vi "ZVisualize.vi"() -> ()   [LabVIEW 2016]
uses:
  subVI/ZDataVIS_StateWire.ctl
  <vilib>/Utility/miscctls.llb/LVPointDoubleTypeDef.ctl
panel:
  in  "update":bool
  out "Field":dbl=4.108108108108109
  out "slowest":dbl=7.00003046875
  in  "e^2/h?":bool
  out "X line cut":cluster{"Vfast":dbl[], dbl[]}(graph)
  out "Y line cut":cluster{"Vfast":dbl[], dbl[]}(graph)
  in  "Y Axis":T1(ring)=enum."dI/dV 2T"
  out "XY Graph":cluster{dbl[], dbl[]}(graph)
  out "Comments":string
  in  "X Scale Selection":enum32{"Manual", "Auto"}(tab)=enum."Auto"
  in  "Manual CTLs":T2={"X Low"=-0.2, "X High"=-0.1, "X Step Size"=0.001} {"X Step Size" format="%#_6p"; "X High" format="%#_6p"; "X Low" format="%#_6p"}
  in  "Auto CTLs":cluster{"METHOD":bool, "Steps":dbl}={"METHOD"=FALSE, "Steps"=100.0}
  out "2term Intensity":dbl[][](graph)
  in  "X Axis":T1(ring)=enum."dI/dV 2T"
  in  "Z Axis":T1(ring)
  in  "Fake Point Value":dbl format="%#_13g"
  in  "Filter retrieved data? 2":bool=TRUE
  in  "side points 4T 2":i32=8
  out "side points 4Ttemp":i32=8
  in  "side points 2T 2":i32=12
  out "side points 2Ttemp":i32=12
  in  "side points 4T":i32=8
  in  "side points 2T":i32=12
  in  "Fit Points 2":dbl=10.0
  in  "T/B     third axis":bool
  in  "color scale":u32[](array[colorbox])=[16711680, 16772608, 6618880, 3381759, 16860, 10420479]
  in  "Voffset -2T":dbl=2e-05 format="%#_6p"
  in  "Voffset-4T":dbl=-5e-05 format="%#_4p"
  in  "Field/Temperature":i32(slide) min=0 max=36 step=1
  out "Scan names":string[](array[string])=["DAQ_Vbg", "B", "B"]
  out "Cursor Graph":cluster{dbl[], dbl[]}(graph)={[0.0, 0.0, 0.0, 0.0, 0.0, 0.0, 0.0, 0.0, 0.25, 0.25, 0.25, 0.25, 0.25, 0.25, 0.25, 0.25, 0.5, 0.5, 0.5, 0.5, 0.5, 0.5, 0.5, 0.5, 0.75, 0.75, 0.75, 0.75, 0.75, 0.75, 0.75, 0.75, 1.0, 1.0, 1.0, 1.0, 1.0, 1.0, 1.0, 1.0, 1.25, 1.25, 1.25, 1.25, 1.25, 1.25, 1.25, 1.25, 1.5, 1.5, 1.5, 1.5, 1.5, 1.5, 1.5, 1.5, 1.75, 1.75, 1.75, 1.75, 1.75, 1.75, 1.75, 1.75, 2.0, 2.0, 2.0, 2.0, 2.0, 2.0, 2.0, 2.0, 2.25, 2.25, 2.25, 2.25, 2.25, 2.25, 2.25, 2.25, 2.5, 2.5, 2.5, 2.5, 2.5, 2.5, 2.5, 2.5, 2.75, 2.75, 2.75, 2.75, 2.75, 2.75, 2.75, 2.75, 3.0, 3.0, 3.0, 3.0, 3.0, 3.0, 3.0, 3.0, 3.25, 3.25, 3.25, 3.25, 3.25, 3.25, 3.25, 3.25, 3.5, 3.5, 3.5, 3.5, 3.5, 3.5, 3.5, 3.5, 3.75, 3.75, 3.75, 3.75, 3.75, 3.75, 3.75, 3.75, 4.0, 4.0, 4.0, 4.0, 4.0, 4.0, 4.0, 4.0, 4.25, 4.25, 4.25, 4.25, 4.25, 4.25, 4.25, 4.25, 4.5, 4.5, 4.5, 4.5, 4.5, 4.5, 4.5, 4.5, 4.75, 4.75, 4.75, 4.75, 4.75, 4.75, 4.75, 4.75, 5.0, 5.0, 5.0, 5.0, 5.0, 5.0, 5.0, 5.0, 5.25, 5.25, 5.25, 5.25, 5.25, 5.25, 5.25, 5.25, 5.5, 5.5, 5.5, 5.5, 5.5, 5.5, 5.5, 5.5, 5.75, 5.75, 5.75, 5.75, 5.75, 5.75, 5.75, 5.75, 6.0, 6.0, 6.0, 6.0, 6.0, 6.0, 6.0, 6.0, 6.25, 6.25, 6.25, 6.25, 6.25, 6.25, 6.25, 6.25, 6.5, 6.5, 6.5, 6.5, 6.5, 6.5, 6.5, 6.5, 6.75, 6.75, 6.75, 6.75, 6.75, 6.75, 6.75, 6.75, 7.0, 7.0, 7.0, 7.0, 7.0, 7.0, 7.0, 7.0, 7.25, 7.25, 7.25, 7.25, 7.25, 7.25, 7.25, 7.25, 7.5, 7.5, 7.5, 7.5, 7.5, 7.5, 7.5, 7.5, 7.75, 7.75, 7.75, 7.75, 7.75, 7.75, 7.75, 7.75, 8.0, 8.0, 8.0, 8.0, 8.0, 8.0, 8.0, 8.0, 8.25, 8.25, 8.25, 8.25, 8.25, 8.25, 8.25, 8.25, 8.5, 8.5, 8.5, 8.5, 8.5, 8.5, 8.5, 8.5, 8.75, 8.75, 8.75, 8.75, 8.75, 8.75, 8.75, 8.75, 9.0, 9.0, 9.0, 9.0, 9.0, 9.0, 9.0, 9.0, 9.25, 9.25, 9.25, 9.25, 9.25, 9.25, 9.25, 9.25, 9.5, 9.5, 9.5, 9.5, 9.5, 9.5, 9.5, 9.5, 9.75, 9.75, 9.75, 9.75, 9.75, 9.75, 9.75, 9.75, 10.0, 10.0, 10.0, 10.0, 10.0, 10.0, 10.0, 10.0, 10.25, 10.25, 10.25, 10.25, 10.25, 10.25, 10.25, 10.25, 10.5, 10.5, 10.5, 10.5, 10.5, 10.5, 10.5, 10.5, 10.75, 10.75, 10.75, 10.75, 10.75, 10.75, 10.75, 10.75, 11.0, 11.0, 11.0, 11.0, 11.0, 11.0, 11.0, 11.0, 11.25, 11.25, 11.25, 11.25, 11.25, 11.25, 11.25, 11.25, 11.5, 11.5, 11.5, 11.5, 11.5, 11.5, 11.5, 11.5, 11.75, 11.75, 11.75, 11.75, 11.75, 11.75, 11.75, 11.75, 12.0, 12.0, 12.0, 12.0, 12.0, 12.0, 12.0, 12.0, 12.25, 12.25, 12.25, 12.25, 12.25, 12.25, 12.25, 12.25, 12.5, 12.5, 12.5, 12.5, 12.5, 12.5, 12.5, 12.5, 12.75, 12.75, 12.75, 12.75, 12.75, 12.75, 12.75, 12.75, 13.0, 13.0, 13.0, 13.0, 13.0, 13.0, 13.0, 13.0, 13.25, 13.25, 13.25, 13.25, 13.25, 13.25, 13.25, 13.25, 13.5, 13.5, 13.5, 13.5, 13.5, 13.5, 13.5, 13.5, 13.75, 13.75, 13.75, 13.75, 13.75, 13.75, 13.75, 13.75, 14.0, 14.0, 14.0, 14.0, 14.0, 14.0, 14.0, 14.0, 14.25, 14.25, 14.25, 14.25, 14.25, 14.25, 14.25, 14.25, 14.5, 14.5, 14.5, 14.5, 14.5, 14.5, 14.5, 14.5, 14.75, 14.75, 14.75, 14.75, 14.75, 14.75, 14.75, 14.75, 15.0, 15.0, 15.0, 15.0, 15.0, 15.0, 15.0, 15.0], [0.0, 1.0, 2.0, 3.0, 4.0, 5.0, 6.0, 7.0, 0.0, 1.0, 2.0, 3.0, 4.0, 5.0, 6.0, 7.0, 0.0, 1.0, 2.0, 3.0, 4.0, 5.0, 6.0, 7.0, 0.0, 1.0, 2.0, 3.0, 4.0, 5.0, 6.0, 7.0, 0.0, 1.0, 2.0, 3.0, 4.0, 5.0, 6.0, 7.0, 0.0, 1.0, 2.0, 3.0, 4.0, 5.0, 6.0, 7.0, 0.0, 1.0, 2.0, 3.0, 4.0, 5.0, 6.0, 7.0, 0.0, 1.0, 2.0, 3.0, 4.0, 5.0, 6.0, 7.0, 0.0, 1.0, 2.0, 3.0, 4.0, 5.0, 6.0, 7.0, 0.0, 1.0, 2.0, 3.0, 4.0, 5.0, 6.0, 7.0, 0.0, 1.0, 2.0, 3.0, 4.0, 5.0, 6.0, 7.0, 0.0, 1.0, 2.0, 3.0, 4.0, 5.0, 6.0, 7.0, 0.0, 1.0, 2.0, 3.0, 4.0, 5.0, 6.0, 7.0, 0.0, 1.0, 2.0, 3.0, 4.0, 5.0, 6.0, 7.0, 0.0, 1.0, 2.0, 3.0, 4.0, 5.0, 6.0, 7.0, 0.0, 1.0, 2.0, 3.0, 4.0, 5.0, 6.0, 7.0, 0.0, 1.0, 2.0, 3.0, 4.0, 5.0, 6.0, 7.0, 0.0, 1.0, 2.0, 3.0, 4.0, 5.0, 6.0, 7.0, 0.0, 1.0, 2.0, 3.0, 4.0, 5.0, 6.0, 7.0, 0.0, 1.0, 2.0, 3.0, 4.0, 5.0, 6.0, 7.0, 0.0, 1.0, 2.0, 3.0, 4.0, 5.0, 6.0, 7.0, 0.0, 1.0, 2.0, 3.0, 4.0, 5.0, 6.0, 7.0, 0.0, 1.0, 2.0, 3.0, 4.0, 5.0, 6.0, 7.0, 0.0, 1.0, 2.0, 3.0, 4.0, 5.0, 6.0, 7.0, 0.0, 1.0, 2.0, 3.0, 4.0, 5.0, 6.0, 7.0, 0.0, 1.0, 2.0, 3.0, 4.0, 5.0, 6.0, 7.0, 0.0, 1.0, 2.0, 3.0, 4.0, 5.0, 6.0, 7.0, 0.0, 1.0, 2.0, 3.0, 4.0, 5.0, 6.0, 7.0, 0.0, 1.0, 2.0, 3.0, 4.0, 5.0, 6.0, 7.0, 0.0, 1.0, 2.0, 3.0, 4.0, 5.0, 6.0, 7.0, 0.0, 1.0, 2.0, 3.0, 4.0, 5.0, 6.0, 7.0, 0.0, 1.0, 2.0, 3.0, 4.0, 5.0, 6.0, 7.0, 0.0, 1.0, 2.0, 3.0, 4.0, 5.0, 6.0, 7.0, 0.0, 1.0, 2.0, 3.0, 4.0, 5.0, 6.0, 7.0, 0.0, 1.0, 2.0, 3.0, 4.0, 5.0, 6.0, 7.0, 0.0, 1.0, 2.0, 3.0, 4.0, 5.0, 6.0, 7.0, 0.0, 1.0, 2.0, 3.0, 4.0, 5.0, 6.0, 7.0, 0.0, 1.0, 2.0, 3.0, 4.0, 5.0, 6.0, 7.0, 0.0, 1.0, 2.0, 3.0, 4.0, 5.0, 6.0, 7.0, 0.0, 1.0, 2.0, 3.0, 4.0, 5.0, 6.0, 7.0, 0.0, 1.0, 2.0, 3.0, 4.0, 5.0, 6.0, 7.0, 0.0, 1.0, 2.0, 3.0, 4.0, 5.0, 6.0, 7.0, 0.0, 1.0, 2.0, 3.0, 4.0, 5.0, 6.0, 7.0, 0.0, 1.0, 2.0, 3.0, 4.0, 5.0, 6.0, 7.0, 0.0, 1.0, 2.0, 3.0, 4.0, 5.0, 6.0, 7.0, 0.0, 1.0, 2.0, 3.0, 4.0, 5.0, 6.0, 7.0, 0.0, 1.0, 2.0, 3.0, 4.0, 5.0, 6.0, 7.0, 0.0, 1.0, 2.0, 3.0, 4.0, 5.0, 6.0, 7.0, 0.0, 1.0, 2.0, 3.0, 4.0, 5.0, 6.0, 7.0, 0.0, 1.0, 2.0, 3.0, 4.0, 5.0, 6.0, 7.0, 0.0, 1.0, 2.0, 3.0, 4.0, 5.0, 6.0, 7.0, 0.0, 1.0, 2.0, 3.0, 4.0, 5.0, 6.0, 7.0, 0.0, 1.0, 2.0, 3.0, 4.0, 5.0, 6.0, 7.0, 0.0, 1.0, 2.0, 3.0, 4.0, 5.0, 6.0, 7.0, 0.0, 1.0, 2.0, 3.0, 4.0, 5.0, 6.0, 7.0, 0.0, 1.0, 2.0, 3.0, 4.0, 5.0, 6.0, 7.0, 0.0, 1.0, 2.0, 3.0, 4.0, 5.0, 6.0, 7.0, 0.0, 1.0, 2.0, 3.0, 4.0, 5.0, 6.0, 7.0, 0.0, 1.0, 2.0, 3.0, 4.0, 5.0, 6.0, 7.0, 0.0, 1.0, 2.0, 3.0, 4.0, 5.0, 6.0, 7.0, 0.0, 1.0, 2.0, 3.0, 4.0, 5.0, 6.0, 7.0]}
  in  "Fit Points":dbl=10.0
  in  "file path (use dialog)":path=path "B:/SketchSET/SA03008H.20180718/processed/51-B+BG_0to15_0.25steps_@0-7T_1step_at.2Hz.dat"
  in  "OK":bool
  # "Y not implemented"
  # "End"
  # "Start"
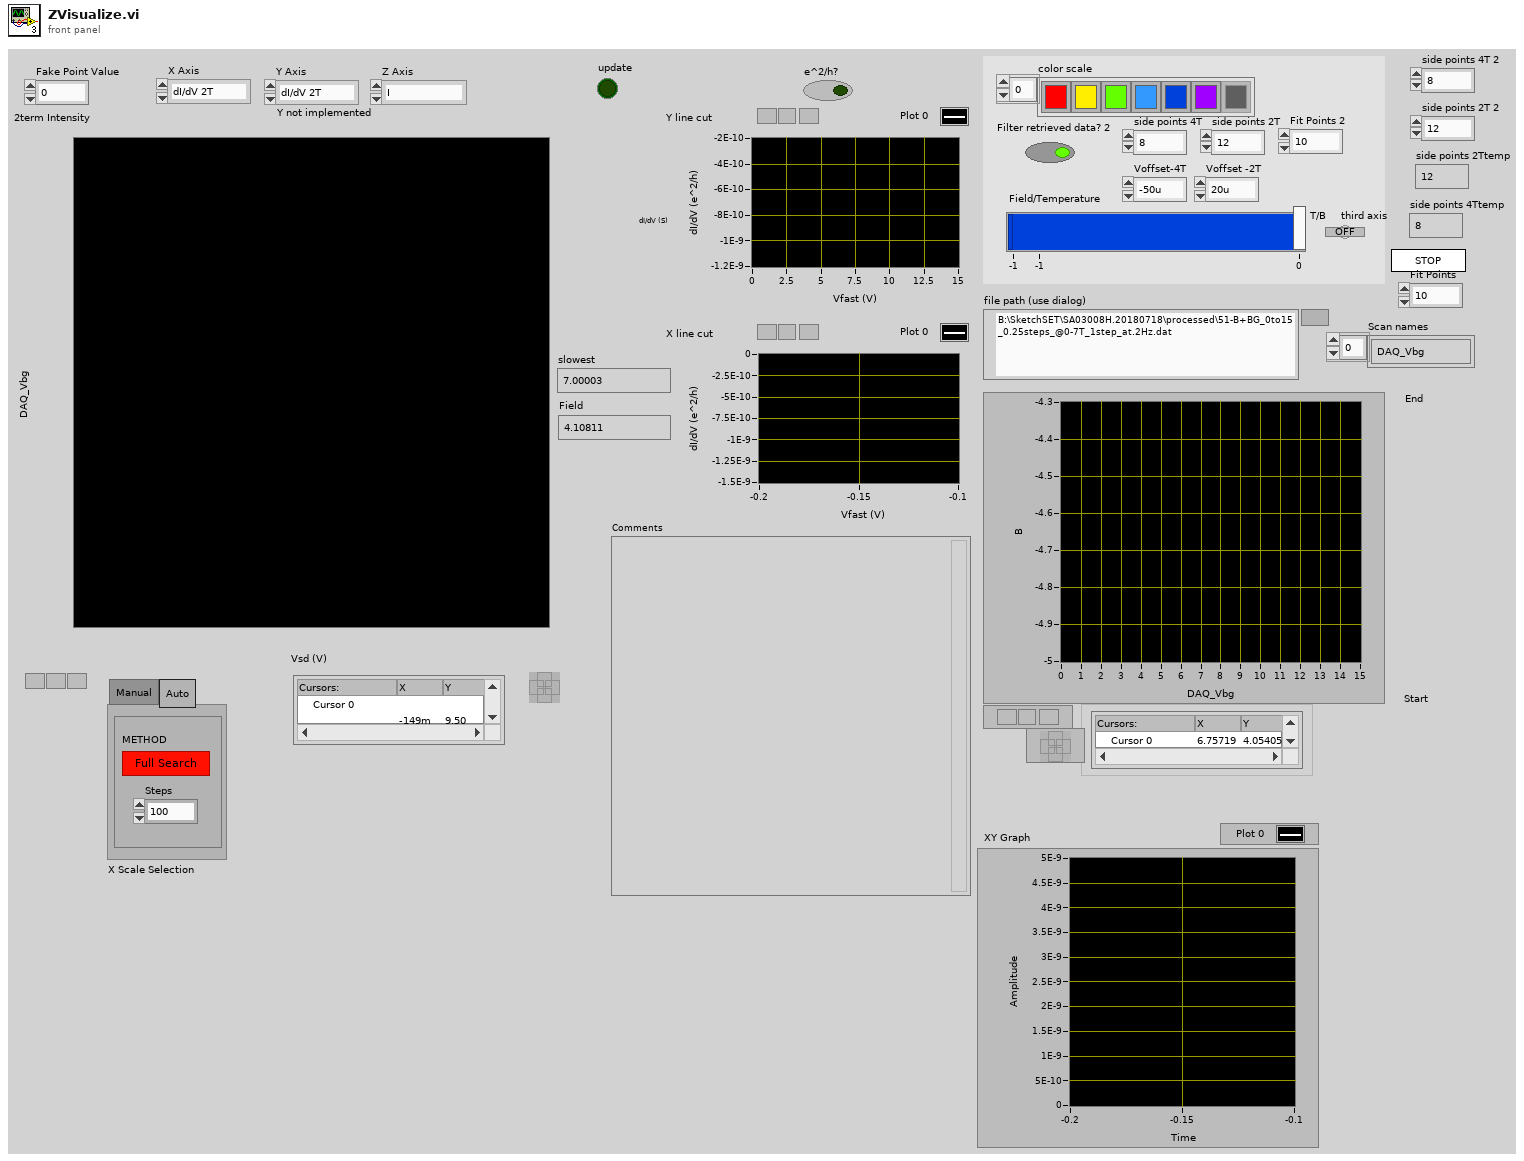
[diagram p1: front panel]
types:
  T1 = enum16{"I", "Vsd", "V4T", "dI/dV 2T", "dV/dI 2T", "dV/dI 4T", "dI/dV 4T"}
  T2 = cluster{"X Low":dbl, "X High":dbl, "X Step Size":dbl}
  T3 = enum32{"invalid app kind", "Development System", "Run Time System", "Student Edition", "Embedded LabVIEW", "Evaluation", "Custom"}
  T4 = cluster{"I":dbl[], "Vsd":dbl[], "V4T":dbl[], "dI/dV 2T":dbl[], "dV/dI 2T":dbl[], "dV/dI 4T":dbl[], "dI/dV 4T":dbl[]}[][][]
  T5 = enum32{"Invalid", "Standard", "Closed", "Hidden", "Minimized", "Maximized"}
  T6 = typedef "ZDataVIS_StateWire.ctl" = cluster{"Core":cluster{"Current VI Reference":refnum<vi>, "Close Panel on Exit?":bool}, "Sweep Data Cluster":cluster{"Vfast":dbl[][], "Vslow":dbl[], "Vslowest":dbl[], "Comments":string, "Scan names":string[]}, "Cursor Info":cluster{"Fast Index":dbl[], "Slow Index":dbl, "Slow Indices":dbl[], "Raw Cursor Position":T7, "Field / temp":i32}, "Scan names":string[], "Data DVR":refnum<data-value>}
  T7 = typedef "LVPointDoubleTypeDef.ctl" = cluster{"X":dbl, "Y":dbl}
  T8 = cluster{"Fast Index (Cursor X)":dbl[], "Slow Index (Cursor Y)":dbl, "Slow Indices":dbl[], "Raw Cursor Position":T7}
  T9 = cluster{"Vfast":dbl[][], "Vslow":dbl[], "Vslowest":dbl[], "Comments":string, "Scan names":string[]}
  T10 = cluster{"Current VI Reference":refnum<vi>, "Close Panel on Exit?":bool}
  T11 = cluster{"IV":cluster{dbl[], dbl[]}[][][], "IV-2T":cluster{dbl[], dbl[]}[][][], "Vfast":dbl[][], "Vslow":dbl[], "Vslowest":dbl[], "Comments":string, "Scan names":string[]}[]
  T12 = cluster{"IV":cluster{dbl[], dbl[]}[][][], "IV-2T":cluster{dbl[], dbl[]}[][][], "Vfast":dbl[][], "Vslow":dbl[], "Vslowest":dbl[], "Comments":string, "Scan names":string[]}
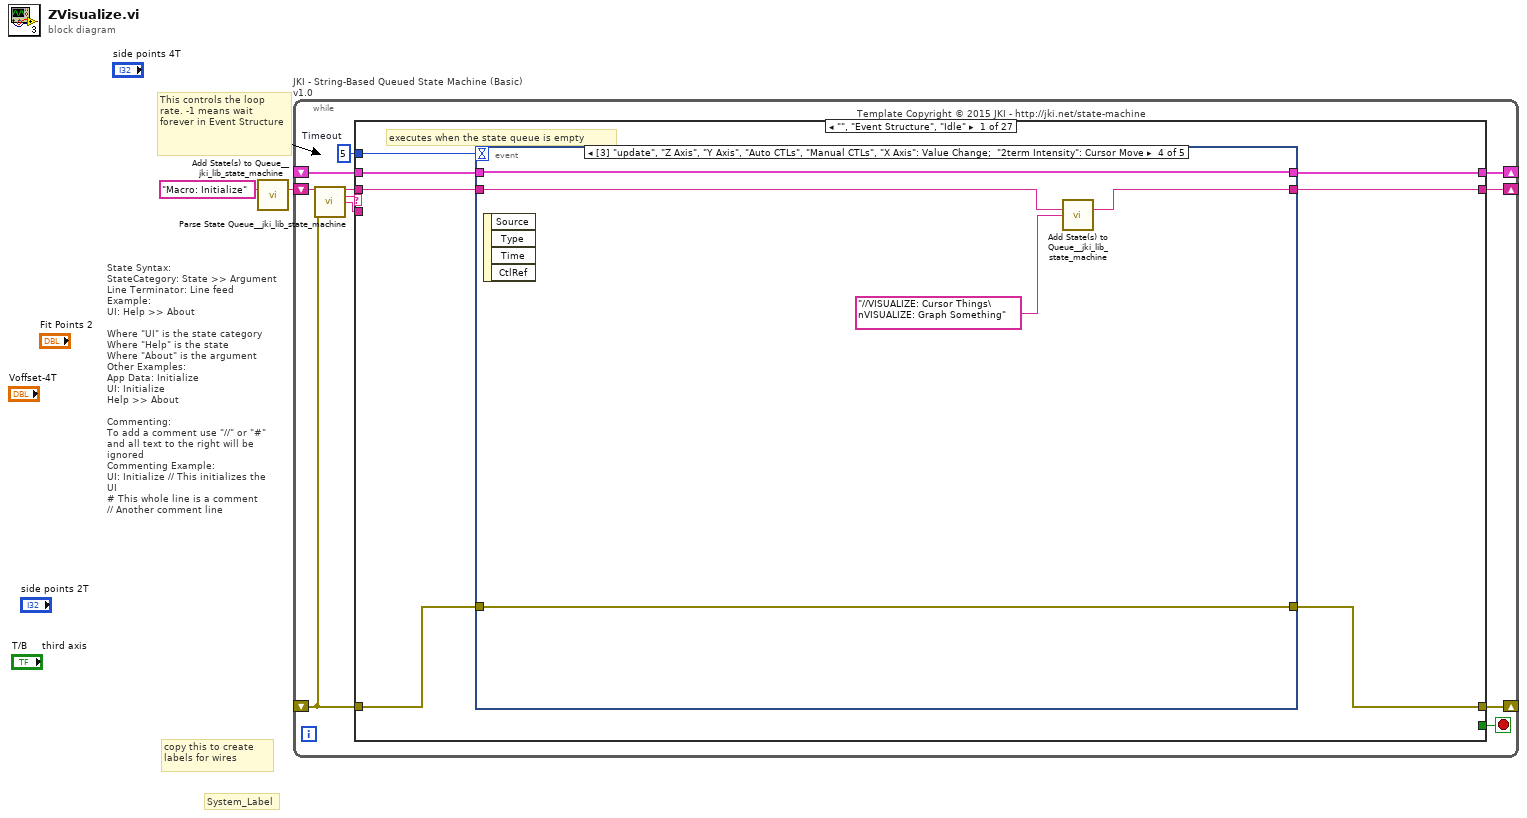
[diagram p0: block diagram]
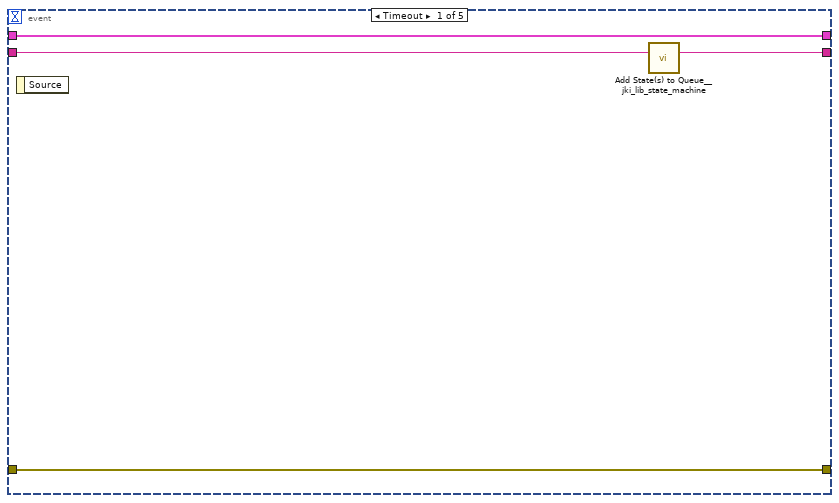
[diagram p2: hidden frame]
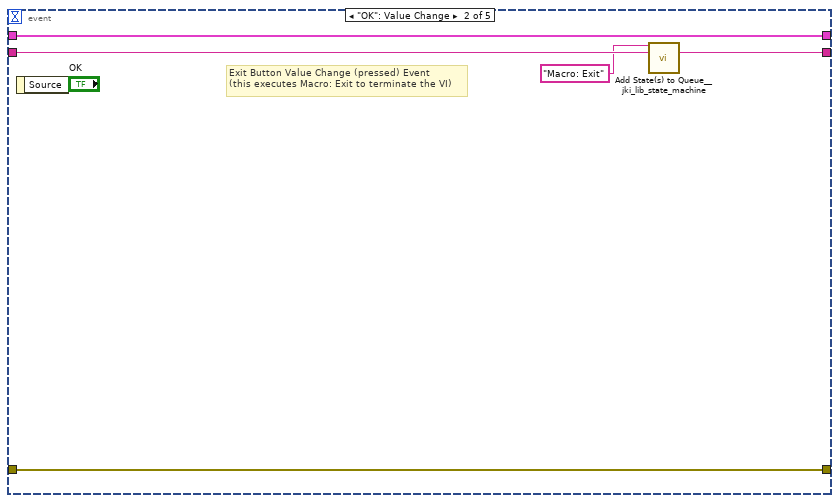
[diagram p3: hidden frame]
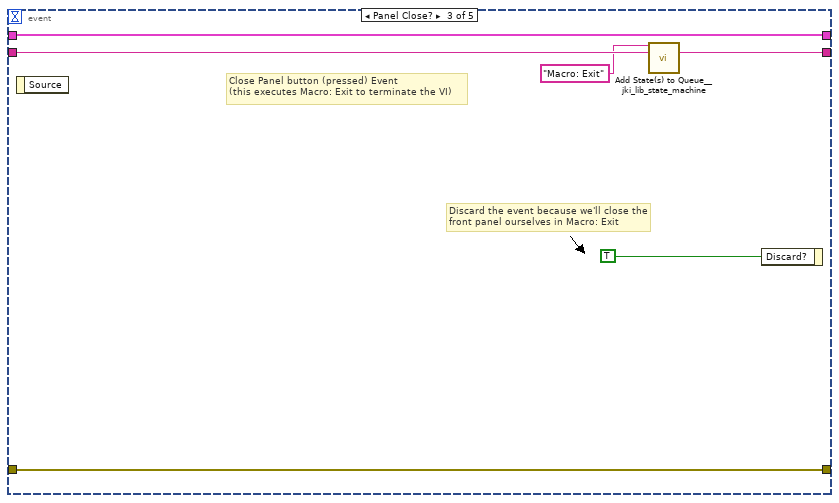
[diagram p4: hidden frame]
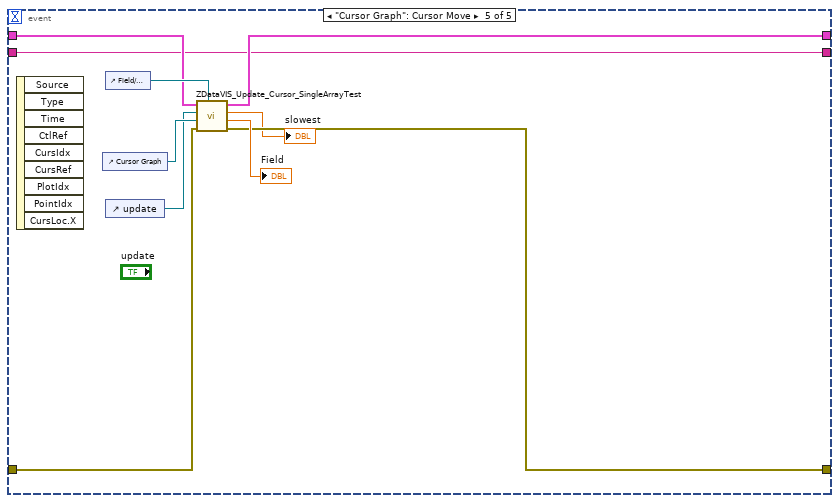
[diagram p5: hidden frame]
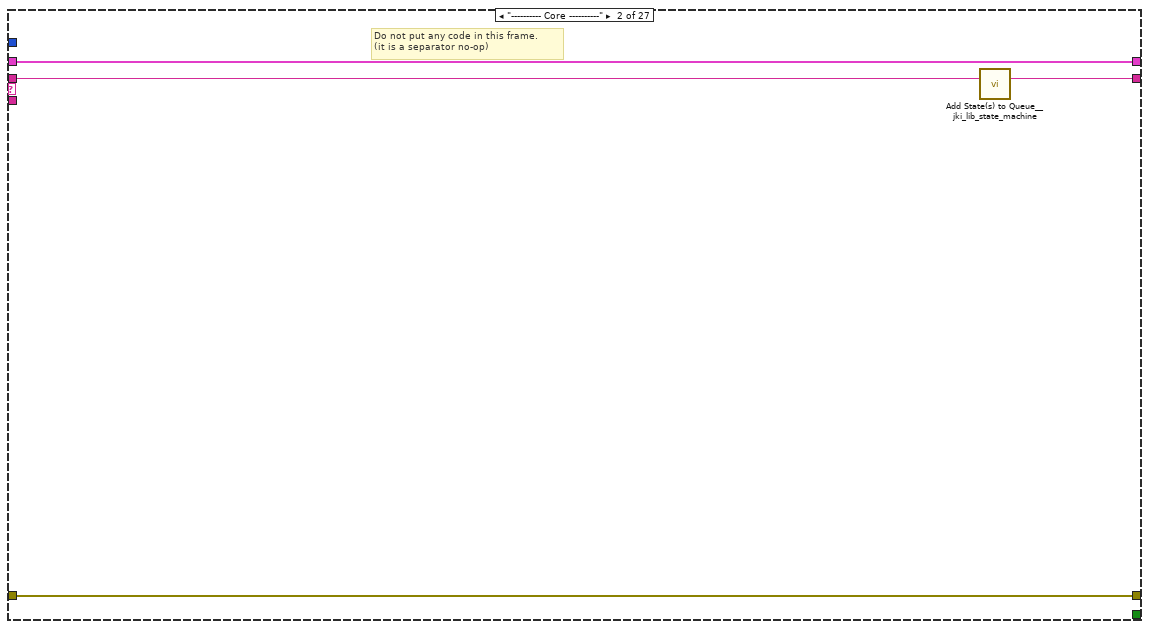
[diagram p6: hidden frame]
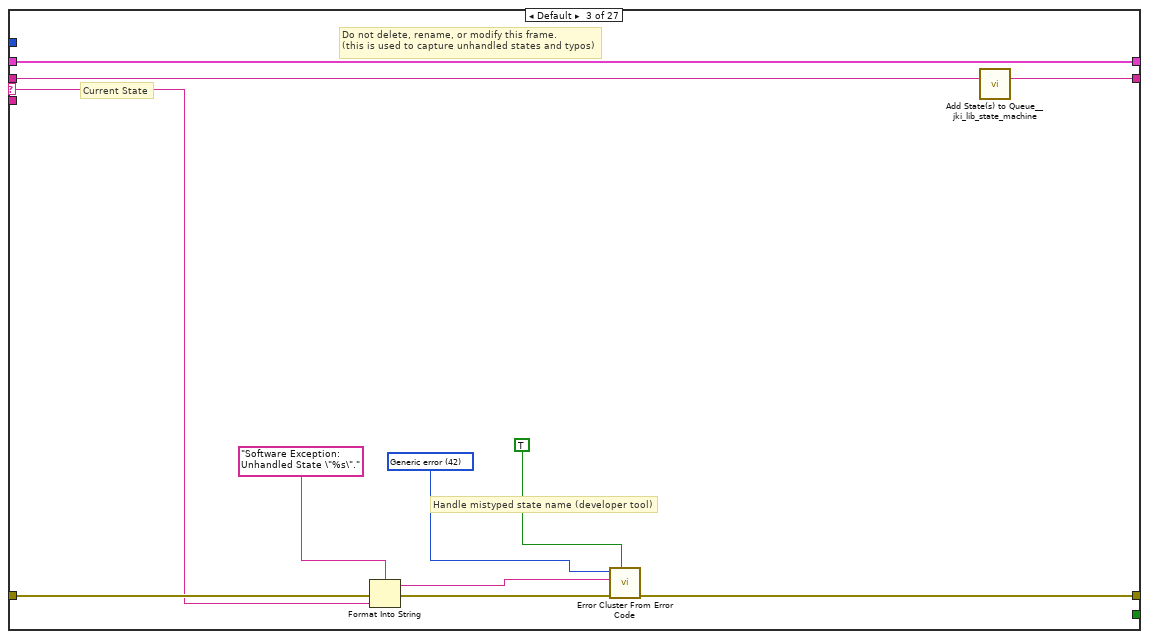
[diagram p7: hidden frame]
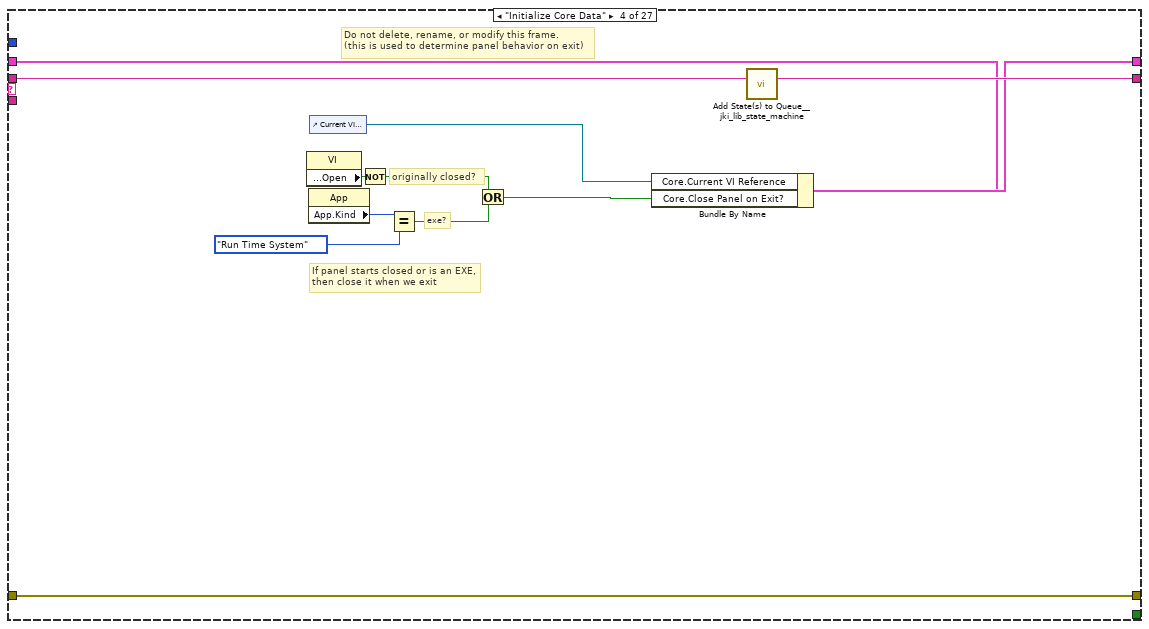
[diagram p8: hidden frame]
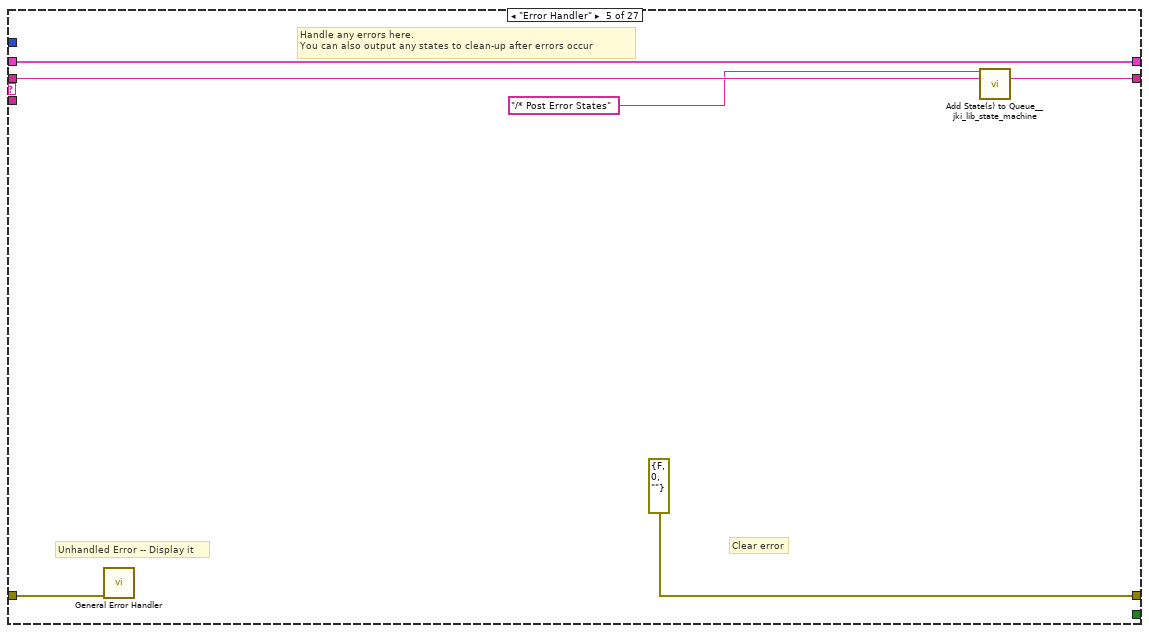
[diagram p9: hidden frame]
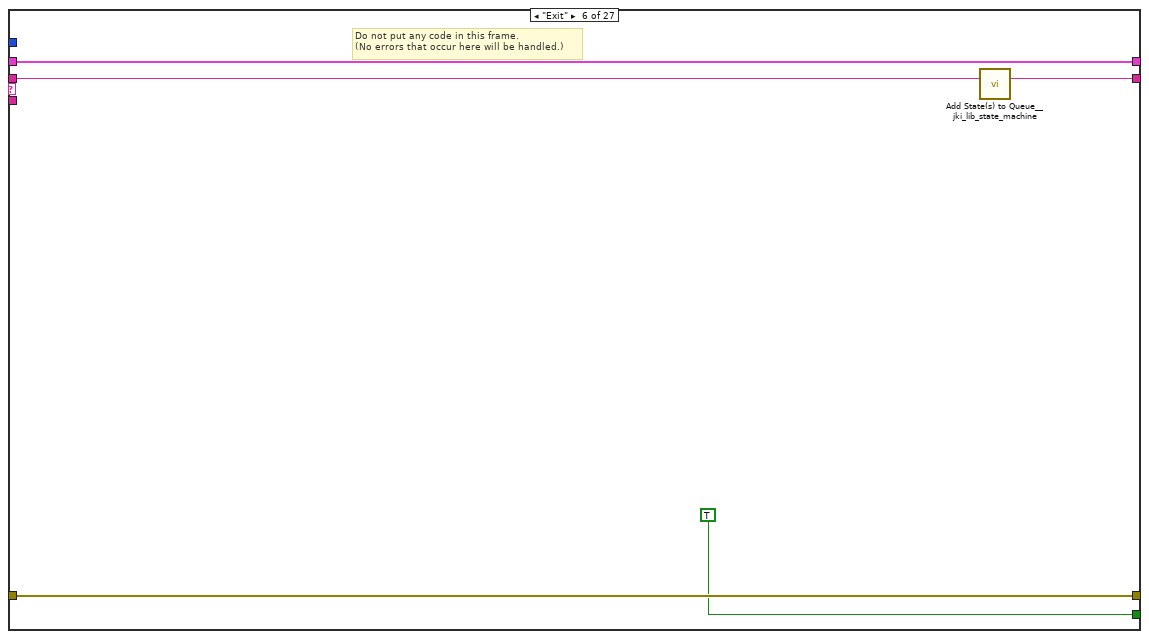
[diagram p10: hidden frame]
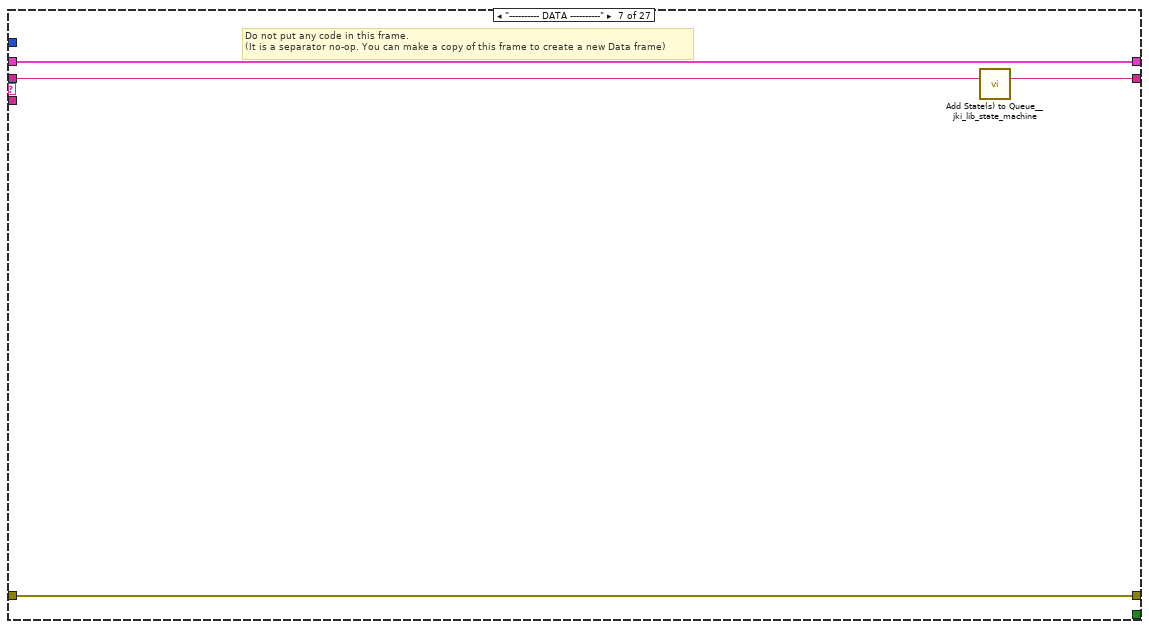
[diagram p11: hidden frame]
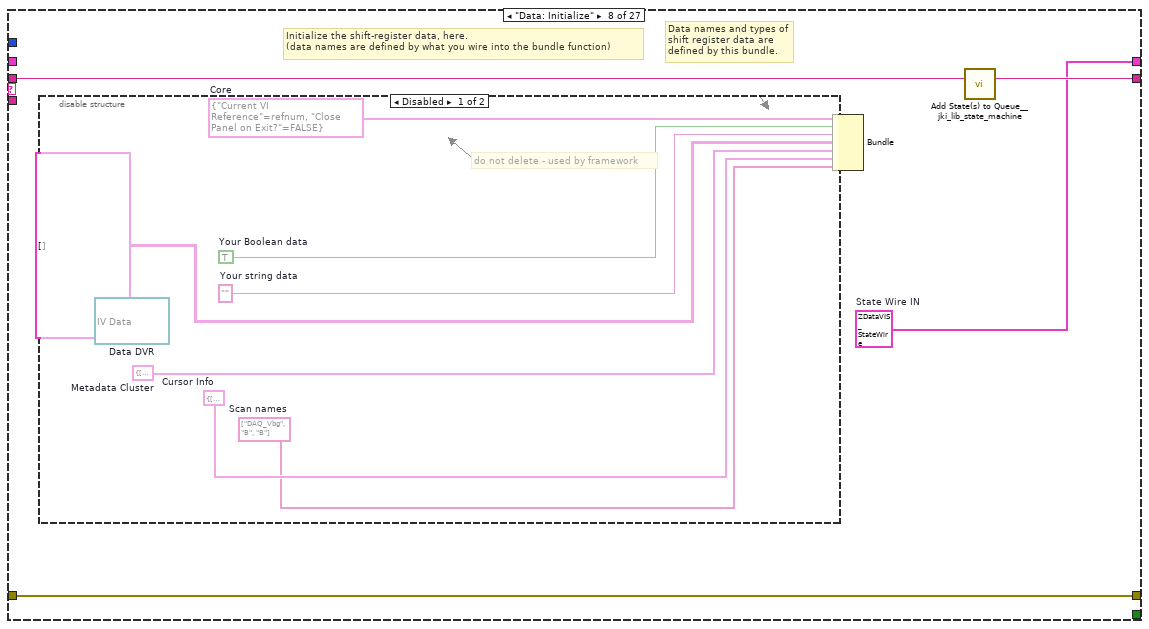
[diagram p12: hidden frame]
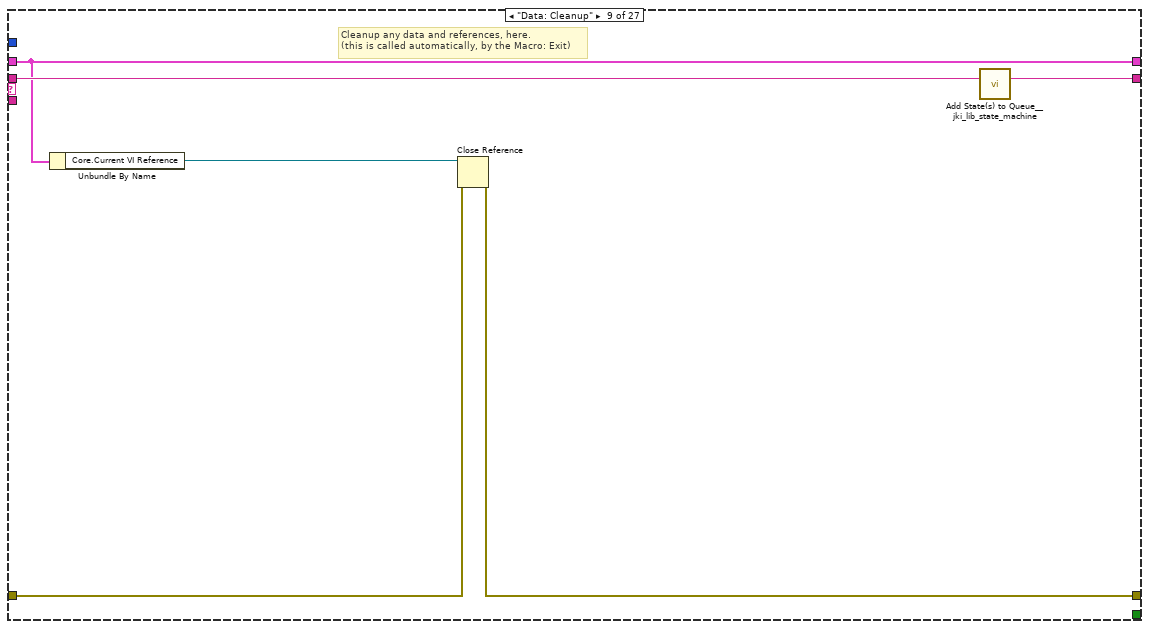
[diagram p14: hidden frame]
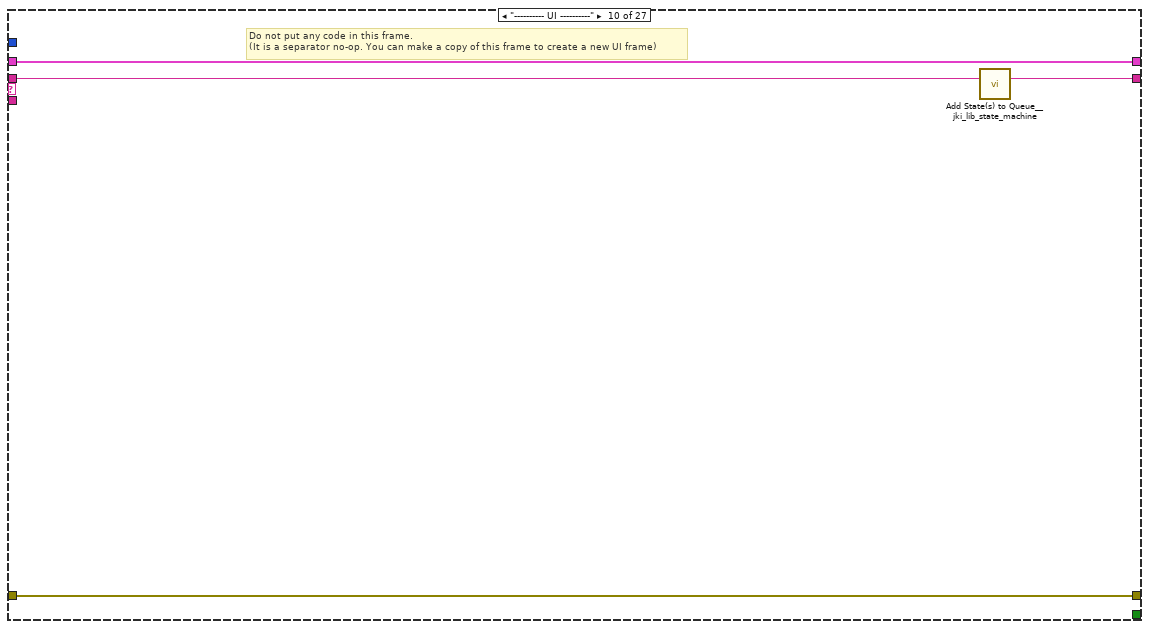
[diagram p15: hidden frame]
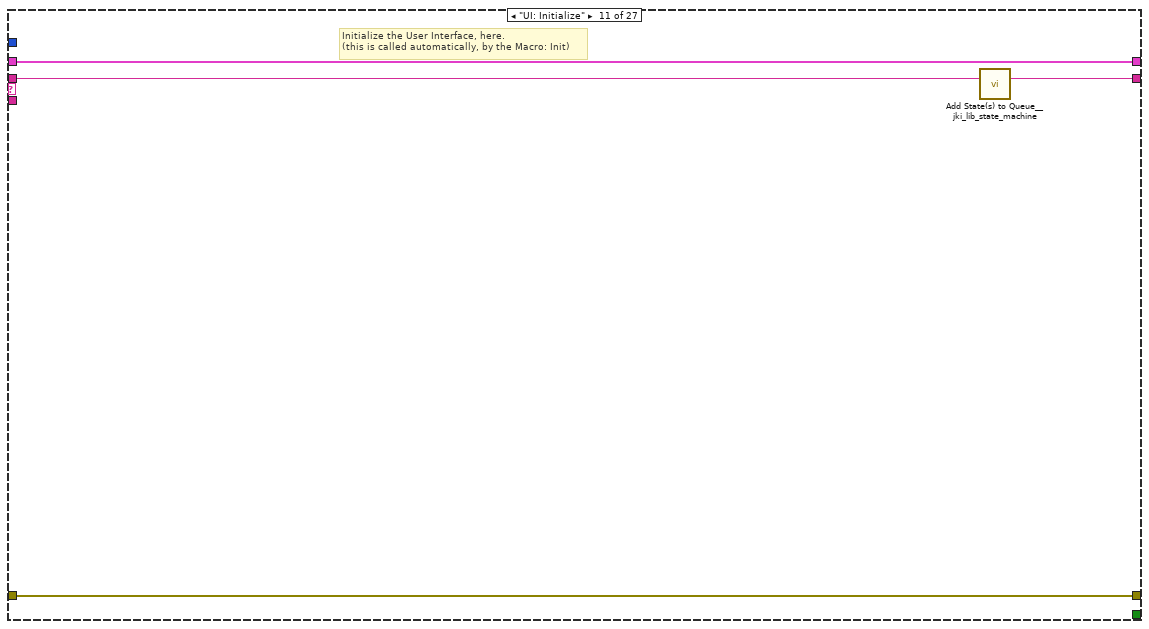
[diagram p16: hidden frame]
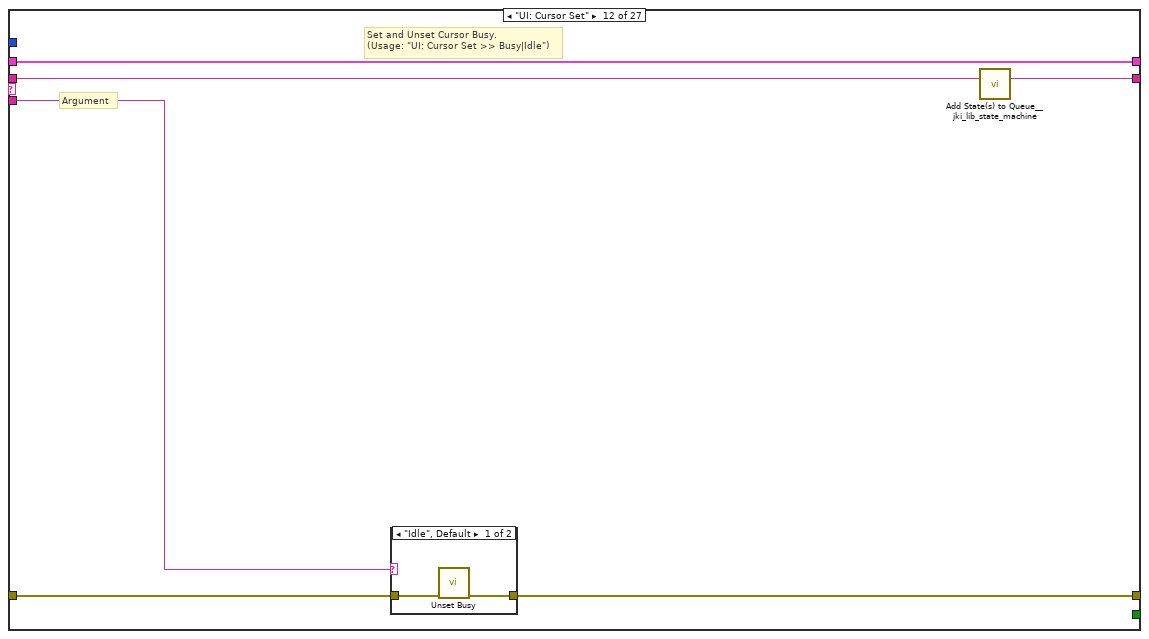
[diagram p17: hidden frame]
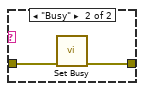
[diagram p18: hidden frame]
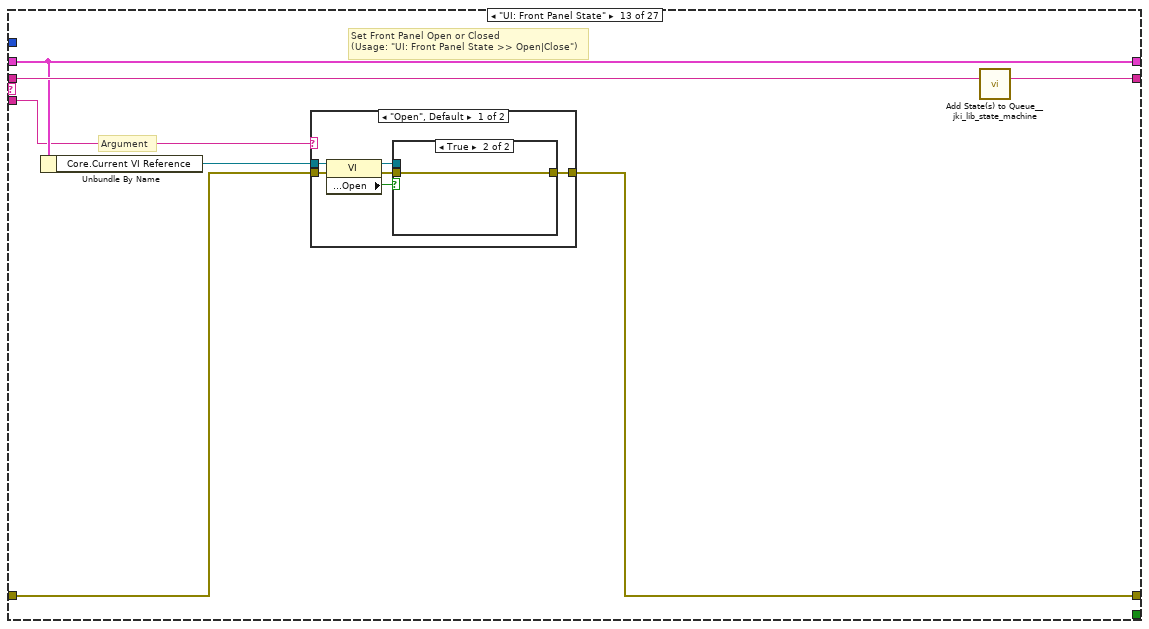
[diagram p19: hidden frame]
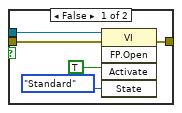
[diagram p20: hidden frame]
diagram:
  # "State Syntax:\nStateCategory: State >> Argument\nLine Terminator: Line feed\nExample:\nUI: Help >> About\n\nWhere \"UI\" is the state category\nWhere \"Help\" is the state\nWhere \"About\" is the argument\nOther Examples:\nApp Data: Initialize\nUI: Initialize\nHelp >> About\n\nCommenting:\nTo add a comment use \"//\" or \"#\" and all text to the right will be ignored\nCommenting Example:\nUI: Initialize // This initializes the UI\n# This whole line is a comment\n// Another comment line"
  # "copy this to create labels for wires"
  # "This controls the loop rate. -1 means wait forever in Event Structure"
  # "System_Label"
  n1 = call <vilib>:"Add State(s) to Queue__jki_lib_state_machine.vi"("State(s) in (\"\")"="Macro: Initialize") -> ("States Out"=w2:string)  [unwired: 14 in]
  n2 = while "JKI - String-Based Queued State Machine (Basic) v1.0" {
    shift-right: [w6] -> _
    shift-left: _ -> [w5]
    shift-right: [w9] -> _
    shift-left: _ -> [w3]
    shift-right: [w8] -> _
    shift-left: w2 -> [w10]
    stop <- w7 stop-if-true
    w4 = 5  # Timeout
    # "Template Copyright © 2015 JKI - http://jki.net/state-machine"
    n3 = call <vilib>:"Parse State Queue__jki_lib_state_machine.vi"("State Queue"=w10, "Error In (no error)"=w3) -> ("Remaining States"=w12:string, "Current State"=w13:string, "Arguments"=w11:string)  [unwired: 11 in]
    n4 = case shown="\"\", \"Event Structure\", \"Idle\"" w13 {
      selector: w13 -> [_ _ w55 _ _ _ _ _ _ _ _ _ _ _ _ _ _ _ _ _ _ _ _ _ _ _ _]
      tunnel: w12 -> [w20 w54 w59 w77 w83 w88 w92 w96 w109 w113 w117 w123 w134 w160 w165 w175 w180 w191 w195 w217 w221 w225 w243 w257 w261 w273 w305]
      tunnel: w11 -> [_ _ _ _ _ _ _ _ _ _ _ w118 w128 _ _ _ _ _ _ _ _ _ _ _ _ _ _]
      tunnel: w5 -> [w18 w51 w57 w68 w80 w86 w89 _ w104 w110 w115 w121 w130 w157 w162 w172 w177 w188 w192 w211 w218 w222 w241 w254 w258 w263 w306]
      tunnel: [w17 w52 w61 w74 errorcluster {"status"=FALSE, "code"=0, "source"=""} ("error out") w85 w90 w94 w105 w111 w114 w119 w131 w158 w163 w173 w178 w189 w193 w209 w219 w223 w226 w255 w259 w271 w307] -> w9
      tunnel: w3 -> [w16 w52 w60 w74 w79 w85 w90 w94 w106 w111 w114 w120 w132 w158 w163 w173 w178 w189 w193 w214 w219 w223 w227 w255 w259 w271 w308]
      tunnel: [w19 w53 w58 w76 w82 w87 w91 w95 w108 w112 w116 w122 w133 w159 w164 w174 w179 w190 w194 w216 w220 w224 w242 w256 w260 w272 w304] -> w8
      tunnel: [_ _ _ _ _ TRUE _ _ _ _ _ _ _ _ _ _ _ _ _ _ _ _ _ _ _ _ _] -> w7
      tunnel: [w15 w51 w57 w75 w80 w86 w89 w93 w104 w110 w115 w121 w130 w157 w162 w172 w177 w188 w192 w210 w218 w222 w241 w254 w258 w262 w301] -> w6
      tunnel: w4 -> [w14 _ _ _ _ _ _ _ _ _ _ _ _ _ _ _ _ _ _ _ _ _ _ _ _ _ _]
      frame "", "Event Structure", "Idle" {
        # "executes when the state queue is empty"
        n5 = event shown="[3] \"update\", \"Z Axis\", \"Y Axis\", \"Auto CTLs\", \"Manual CTLs\", \"X Axis\": Value Change;  \"2term Intensity\": Cursor Move" {
          selector: _ -> [_ _ _ _ _]
          dyn-events: _ -> [_ _ _ _ _]
          timeout: w14 -> [_ _ _ _ _]
          tunnel: w20 -> [w24 w29 w35 w38 w45]
          tunnel: [w23 w28 w34 w36 w45] -> w19
          tunnel: w18 -> [w21 w26 w32 w40 w47]
          tunnel: [w22 w27 w33 w39 w42] -> w17
          tunnel: w16 -> [w22 w27 w33 w39 w44]
          tunnel: [w21 w26 w32 w40 w46] -> w15
          event Timeout {
            n6 = event-data() -> ()  [unwired: 1 in, 1 out]
            n7 = call <vilib>:"Add State(s) to Queue__jki_lib_state_machine.vi"("State(s) in (\"\")"=w24) -> ("States Out"=w23:string)  [unwired: 14 in]
          }
          event "OK": Value Change {
            # "Exit Button Value Change (pressed) Event\n(this executes Macro: Exit to terminate the VI)"
            n8 = event-data() -> ()  [unwired: 1 in, 1 out]
            n9 = call <vilib>:"Add State(s) to Queue__jki_lib_state_machine.vi"("State(s) in Front (\"\")"="Macro: Exit", "State(s) in (\"\")"=w29) -> ("States Out"=w28:string)  [unwired: 13 in]
          }
          event Panel Close? {
            # "Discard the event because we'll close the front panel ourselves in Macro: Exit"
            # "Close Panel button (pressed) Event\n(this executes Macro: Exit to terminate the VI)"
            n10 = event-data() -> ()  [unwired: 1 in, 1 out]
            n11 = call <vilib>:"Add State(s) to Queue__jki_lib_state_machine.vi"("State(s) in Front (\"\")"="Macro: Exit", "State(s) in (\"\")"=w35) -> ("States Out"=w34:string)  [unwired: 13 in]
            n12 = event-data("Discard?"=TRUE) -> ()  [unwired: 1 in, 1 out]
          }
          event "update", "Z Axis", "Y Axis", "Auto CTLs", "Manual CTLs", "X Axis": Value Change; "2term Intensity": Cursor Move {
            n13 = event-data() -> ()  [unwired: 1 in, 4 out]
            n14 = call <vilib>:"Add State(s) to Queue__jki_lib_state_machine.vi"("State(s) in (\"\")"=w38, "State(s) at Back (\"\")"="//VISUALIZE: Cursor Things\nVISUALIZE: Graph Something" ("State(s) at Back (\"\")")) -> ("States Out"=w36:string)  [unwired: 13 in]
          }
          event "Cursor Graph": Cursor Move {
            n15 = event-data() -> ()  [unwired: 1 in, 9 out]
            n16 = control-ref of="Cursor Graph"() -> (w49:refnum<vi>)
            n17 = control-ref of="Field/Temperature"() -> (w48:refnum<vi>)
            n18 = control-ref of="update"() -> (w43:refnum<vi>)
            n19 = call "ZDataVIS_Update_Cursor_SingleArrayTest.vi"("Field/Temperature 2"=w48, "error in (no error)"=w44, "Cursor Graph"=w49, "update bool"=w43, "State Wire IN 2"=w47) -> ("error out"=w42:errorcluster, "Field"=→"Field":dbl, "slowest"=→"slowest":dbl, "State Wire IN 3"=w46:T6)  [unwired: 3 in]
          }
        }
      }
      frame "---------- Core ----------" {
        # "Do not put any code in this frame.\n(it is a separator no-op)"
        n20 = call <vilib>:"Add State(s) to Queue__jki_lib_state_machine.vi"("State(s) in (\"\")"=w54) -> ("States Out"=w53:string)  [unwired: 14 in]
      }
      frame Default {
        w64 = 42 items=["No error", "Argument error", "Memory is full", "Out of zone", "End of file", "File already open", "Generic file I/O error", "File not found", "File permission error", "Disk is full", "Duplicate path", "Too many files open", "System feature not enabled", "Resource file not found", "Cannot add resource", "Resource not found", "Image not found", "Image memory error", "Pen does not exist", "Config type invalid", "Config token not found", "Config parse error", "Config memory error", "Bad external code format", "Bad external code offset", "External code not present", "Null window", "Destroy window error", "Null menu", "Print aborted", "Bad print record", "Print driver error", "Windows error during printing", "Memory error during printing", "Print dialog error", "Generic print error", "Invalid device refnum", "Device not found", "Device parameter error", "Device unit error", "Cannot open device", "Device call aborted", "Generic error", "Cancelled by user", "Object ID too low", "Object ID too high", "Object not in heap", "Unknown heap", "Unknown object (invalid DefProc)", "Unknown object (DefProc not in table)", "Message out of range", "Invalid (null) method", "Unknown message", "Manager call not supported", "Bad address", "Network operation in progress", "Network operation timed out", "Connection is busy", "Network attribute not supported", "Network error", "Address in use", "System out of memory", "Connection aborted", "Connection refused", "Not connected", "Already connected", "Connection closed", "Initialization error (interapplication manager)", "Bad occurrence", "Wait on unbound occurrence handler", "Occurrence queue overflow", "Datalog type conflict", "Unused", "Unrecognized type (interapplication manager)", "Memory corrupt", "Failed to make temporary DLL", "Old CIN version", "Drag socket not found", "Failed to load drop-object", "Failed to register OLE object", "Failed to release OLE object", "Format specifier type mismatch", "Unknown format specifier", "Too few format specifiers", "Too many format specifiers", "Scan failed", "Newer CIN version", "Error converting to variant", "Runtime menu error", "Password tampered", "Variant attribute not found", "Incompatible variant data type", "Event data is not available", "Event Store is not present", "Occurrence is not found", "Event Queue is not created", "Event info is not available", "Refnum passed is NULL", "Error retrieving Class GUID", "Error retrieving CoClass GUID", "Error retrieving TypeLib GUID.", "Bad built application magic bytes.", "Specific driver is different from the specific driver associated with the Logical Name.", "There is no session opened to the class driver.", "Max Error", "MAX - Error with config objects", "MAX - Error loading configuration", "MAX - Group not supported"]
        # "Current State"
        # "Do not delete, rename, or modify this frame.\n(this is used to capture unhandled states and typos)"
        # "Handle mistyped state name (developer tool)"
        n21 = Format Into String(format string="Software Exception: Unhandled State \"%s\"." ("message"), error in=w60, w55) -> (resulting string=w63:string, error out=w62:errorcluster)  [unwired: 1 in]
        n22 = call <vilib>:"Error Cluster From Error Code.vi"("show call chain? (False)"=TRUE, "error in (no error)"=w62, "error message (\"\")"=w63, "error code (0)"=w64) -> ("error out"=w61:errorcluster)  [unwired: 5 in]
        n23 = call <vilib>:"Add State(s) to Queue__jki_lib_state_machine.vi"("State(s) in (\"\")"=w59) -> ("States Out"=w58:string)  [unwired: 14 in]
      }
      frame "Initialize Core Data" {
        # "Do not delete, rename, or modify this frame.\n(this is used to determine panel behavior on exit)"
        # "originally closed?"
        # "exe?"
        # "If panel starts closed or is an EXE, then close it when we exit"
        n24 = property class="VI"() -> ("Front Panel.Open"=w73:bool)  [unwired: 2 in, 2 out]
        n25 = property class="App"() -> ("App.Kind"=w72:T3)  [unwired: 2 in, 2 out]
        n26 = control-ref of="Current VI Reference"() -> (w66:refnum<vi>)
        n27 = Not(x=w73) -> (.not. x?=w70:bool)
        n28 = Equal?(x=w72, y=T3."Run Time System" ("Application:Kind")) -> (x = y?=w69:bool)
        n29 = Or(x=w70, y=w69) -> (x .or. y?=w67:bool)
        n30 = Bundle By Name(cluster=w68, "Core.Current VI Reference"=w66, "Core.Close Panel on Exit?"=w67) -> (w75:T6)
        n31 = call <vilib>:"Add State(s) to Queue__jki_lib_state_machine.vi"("State(s) in (\"\")"=w77) -> ("States Out"=w76:string)  [unwired: 14 in]
      }
      frame "Error Handler" {
        # "Unhandled Error -- Display it"
        # "Handle any errors here.\nYou can also output any states to clean-up after errors occur"
        # "Clear error"
        n32 = call <vilib>:"General Error Handler.vi"("error in (no error)"=w79) -> ()  [unwired: 10 in, 5 out]
        n33 = call <vilib>:"Add State(s) to Queue__jki_lib_state_machine.vi"("State(s) in Front (\"\")"="/* Post Error States", "State(s) in (\"\")"=w83) -> ("States Out"=w82:string)  [unwired: 13 in]
      }
      frame "Exit" {
        # "Do not put any code in this frame.\n(No errors that occur here will be handled.)"
        n34 = call <vilib>:"Add State(s) to Queue__jki_lib_state_machine.vi"("State(s) in (\"\")"=w88) -> ("States Out"=w87:string)  [unwired: 14 in]
      }
      frame "---------- DATA ----------" {
        # "Do not put any code in this frame.\n(It is a separator no-op. You can make a copy of this frame to create a new Data frame)"
        n35 = call <vilib>:"Add State(s) to Queue__jki_lib_state_machine.vi"("State(s) in (\"\")"=w92) -> ("States Out"=w91:string)  [unwired: 14 in]
      }
      frame "Data: Initialize" {
        w93 = T6 {"Core"={"Current VI Reference"=refnum, "Close Panel on Exit?"=FALSE}, "Sweep Data Cluster"={"Vfast"=[], "Vslow"=[], "Vslowest"=[], "Comments"="", "Scan names"=[]}, "Cursor Info"={"Fast Index"=[], "Slow Index"=0.0, "Slow Indices"=[], "Raw Cursor Position"={"X"=0.0, "Y"=0.0}, "Field / temp"=0}, "Scan names"=[], "Data DVR"=refnum}  # State Wire IN
        # "Data names and types of shift register data are defined by this bundle."
        # "Initialize the shift-register data, here.\n(data names are defined by what you wire into the bundle function)"
        n36 = disable-structure shown="Disabled" {
          frame Disabled {
            w98 = string[] ["DAQ_Vbg", "B", "B"]  # Scan names
            w99 = T8 {"Fast Index (Cursor X)"=[], "Slow Index (Cursor Y)"=0.0, "Slow Indices"=[], "Raw Cursor Position"={"X"=0.0, "Y"=0.0}}  # Cursor Info
            w100 = T9 {"Vfast"=[], "Vslow"=[], "Vslowest"=[], "Comments"="", "Scan names"=[]}  # Metadata Cluster
            (unwired) refnum<data-value> refnum  # Data DVR
            w101 = T10 {"Current VI Reference"=refnum, "Close Panel on Exit?"=FALSE}  # Core
            w102 = ""  # Your string data
            w103 = TRUE  # Your Boolean data
            # "do not delete - used by framework"
            n37 = Bundle("Core"=w101, "Your Boolean data"=w103, "Your string data"=w102, "Data Cell"=T4 [], "Metadata Cluster"=w100, "Cursor Info"=w99, "Scan names"=w98) -> ()  [unwired: 1 in, 1 out]
          }
          frame Enabled {
          }
        }
        n38 = call <vilib>:"Add State(s) to Queue__jki_lib_state_machine.vi"("State(s) in (\"\")"=w96) -> ("States Out"=w95:string)  [unwired: 14 in]
      }
      frame "Data: Cleanup" {
        # "Cleanup any data and references, here.\n(this is called automatically, by the Macro: Exit)"
        n39 = Unbundle By Name(w104) -> ("Core.Current VI Reference"=w107:refnum<vi>)
        n40 = Close Reference(reference=w107, error in (no error)=w106) -> (error out=w105:errorcluster)
        n41 = call <vilib>:"Add State(s) to Queue__jki_lib_state_machine.vi"("State(s) in (\"\")"=w109) -> ("States Out"=w108:string)  [unwired: 14 in]
      }
      frame "---------- UI ----------" {
        # "Do not put any code in this frame.\n(It is a separator no-op. You can make a copy of this frame to create a new UI frame)"
        n42 = call <vilib>:"Add State(s) to Queue__jki_lib_state_machine.vi"("State(s) in (\"\")"=w113) -> ("States Out"=w112:string)  [unwired: 14 in]
      }
      frame "UI: Initialize" {
        # "Initialize the User Interface, here.\n(this is called automatically, by the Macro: Init)"
        n43 = call <vilib>:"Add State(s) to Queue__jki_lib_state_machine.vi"("State(s) in (\"\")"=w117) -> ("States Out"=w116:string)  [unwired: 14 in]
      }
      frame "UI: Cursor Set" {
        # "Argument"
        # "Set and Unset Cursor Busy.\n(Usage: \"UI: Cursor Set >> Busy|Idle\")"
        n44 = case shown="\"Idle\", Default" w118 {
          tunnel: w120 -> [w125 w127]
          tunnel: [w124 w126] -> w119
          frame "Idle", Default {
            n45 = call <vilib>:"Unset Busy.vi"("error in (no error)"=w125) -> ("error out"=w124:errorcluster)  [unwired: 10 in]
          }
          frame "Busy" {
            n46 = call <vilib>:"Set Busy.vi"("error in (no error)"=w127) -> ("error out"=w126:errorcluster)  [unwired: 9 in, 1 out]
          }
        }
        n47 = call <vilib>:"Add State(s) to Queue__jki_lib_state_machine.vi"("State(s) in (\"\")"=w123) -> ("States Out"=w122:string)  [unwired: 14 in]
      }
      frame "UI: Front Panel State" {
        # "Argument"
        # "Set Front Panel Open or Closed\n(Usage: \"UI: Front Panel State >> Open|Close\")"
        n48 = Unbundle By Name(w130) -> ("Core.Current VI Reference"=w129:refnum<vi>)
        n49 = case shown="\"Open\", Default" w128 {
          tunnel: w132 -> [w138 w151]
          tunnel: [w140 w152] -> w131
          tunnel: w129 -> [w139 w149]
          frame "Open", Default {
            n50 = property class="VI"(reference=w139, error in=w138) -> (reference out=w136:refnum<vi>, error out=w137:errorcluster, "Front Panel.Open"=w135:bool)
            n51 = case shown="True" w135 {
              tunnel: [w143 w146] -> w140
              tunnel: w137 -> [w142 w146]
              tunnel: w136 -> [w141 _]
              frame False {
                n52 = invoke class="VI" method="FP.Open"(reference=w141, error in=w142, "Activate"=TRUE, "State"=T5."Standard") -> (error out=w143:errorcluster)  [unwired: 1 in, 4 out]
              }
              frame True {
              }
            }
          }
          frame "Close" {
            n53 = property class="VI"(reference=w149, error in=w151) -> (reference out=w148:refnum<vi>, error out=w150:errorcluster, "Front Panel.Open"=w147:bool)
            n54 = case shown="True" w147 {
              tunnel: [w153 w156] -> w152
              tunnel: w150 -> [w153 w155]
              tunnel: w148 -> [_ w154]
              frame False {
              }
              frame True {
                n55 = invoke class="VI" method="FP.Close"(reference=w154, error in=w155) -> (error out=w156:errorcluster)  [unwired: 1 in, 2 out]
              }
            }
          }
        }
        n56 = call <vilib>:"Add State(s) to Queue__jki_lib_state_machine.vi"("State(s) in (\"\")"=w134) -> ("States Out"=w133:string)  [unwired: 14 in]
      }
      frame "---------- Macro ----------" {
        # "Do not put any code in this frame.\n(It is a separator no-op. You can make a copy of this frame to create a new Macro frame)"
        n57 = call <vilib>:"Add State(s) to Queue__jki_lib_state_machine.vi"("State(s) in (\"\")"=w160) -> ("States Out"=w159:string)  [unwired: 14 in]
      }
      frame "Macro: Initialize" {
        # "Initialization Macro\n(This is called once, when the VI starts)"
        n58 = call <vilib>:"Add State(s) to Queue__jki_lib_state_machine.vi"("State(s) in Front (\"\")"="Data: Initialize\nInitialize Core Data\nUI: Initialize\nUI: Front Panel State >> Open\nMacro: LOAD\nMacro: Visualize", "State(s) in (\"\")"=w165) -> ("States Out"=w164:string)  [unwired: 13 in]
      }
      frame "Macro: Exit" {
        # "Exit Macro\n(This is called once, when the VI exits)"
        n59 = Unbundle By Name(w172) -> ("Core.Close Panel on Exit?"=w171:bool)
        n60 = Select(t="UI: Front Panel State >> Close", s=w171, f="") -> (s? t:f=w168:string)
        n61 = call <vilib>:"Add State(s) to Queue__jki_lib_state_machine.vi"("State(s) in (\"\")"=w168, "State(s) at Back (\"\")"="Data: Cleanup\nExit") -> ("States Out"=w166:string)  [unwired: 13 in]
        n62 = call <vilib>:"Add State(s) to Queue__jki_lib_state_machine.vi"("State(s) in Front (\"\")"=w166, "State(s) in (\"\")"=w175) -> ("States Out"=w174:string)  [unwired: 13 in]
      }
      frame "Macro: LOAD" {
        # "Exit Macro\n(This is called once, when the VI exits)"
        n63 = call <vilib>:"Add State(s) to Queue__jki_lib_state_machine.vi"("State(s) in Front (\"\")"="LOAD: Load that .dat data" ("State(s) in Front (\"\")"), "State(s) in (\"\")"=w180) -> ("States Out"=w179:string)  [unwired: 13 in]
      }
      frame "Macro: VISUALIZE" {
        # "Skip or don't skip filtering step"
        # "Exit Macro\n(This is called once, when the VI exits)"
        n64 = Select(t="VISUALIZE: Apply SG Filter", s="Filter retrieved data? 2", f="") -> (s? t:f=w185:string)
        n65 = call <vilib>:"Add State(s) to Queue__jki_lib_state_machine.vi"("State(s) in Front (\"\")"="VISUALIZE: Initialize Cursor Graph\nVISUALIZE: Initialize Color Tables" ("State(s) in Front (\"\")"), "State(s) in (\"\")"=w185, "State(s) at Back (\"\")"="//VISUALIZE: Cursor Things\nVISUALIZE: Graph Something" ("State(s) at Back (\"\")")) -> ("States Out"=w184:string)  [unwired: 12 in]
        n66 = call <vilib>:"Add State(s) to Queue__jki_lib_state_machine.vi"("State(s) in Front (\"\")"=w184, "State(s) in (\"\")"=w191) -> ("States Out"=w190:string)  [unwired: 13 in]
      }
      frame "---------- LOAD ----------" {
        # "Template Separator\n(You can make a copy of, or modify, this frame)"
        n67 = call <vilib>:"Add State(s) to Queue__jki_lib_state_machine.vi"("State(s) in (\"\")"=w195) -> ("States Out"=w194:string)  [unwired: 14 in]
      }
      frame "LOAD: Load that .dat data" {
        # "DVR"
        # "differentate and rebundle the IV data"
        # "separate meta-ish data and IV data"
        # "Read .dat file"
        n68 = call "DataVIS_Read .DAT Data.vi"("error in (no error)"=w214, "file path (use dialog)"="file path (use dialog)") -> ("error out"=w200:errorcluster, "Array"=w212:T11)  [unwired: 8 in]
        n69 = Index Array(array=w212) -> (element=w213:T12)  [unwired: 1 in]
        n70 = Unbundle By Name(w213) -> ("IV-2T"=w202:cluster{dbl[], dbl[]}[][][], "IV"=w203:cluster{dbl[], dbl[]}[][][], "Vfast"=w208:dbl[][], "Vslow"=w207:dbl[], "Vslowest"=w206:dbl[], "Comments"=w205:string, "Scan names"=w198:string[])
        "Scan names" <- w198
        n71 = Bundle("Vfast"=w208, "Vslow"=w207, "Vslowest"=w206, "Comments"=w205, "Scan names"=w198) -> (w204:T9)  [unwired: 1 in]
        n72 = call "DataVIS_Differentiate_and_Rebundle.vi"("Fit Points"="Fit Points", "error in (no error)"=w200, "IV"=w203, "IV-2T"=w202) -> ("error out"=w199:errorcluster, "Data Cell"=w197:T4)  [unwired: 6 in]
        n73 = New Data Value Reference(data value=w197, error in=w199) -> (data value reference=w196:refnum<data-value>, error out=w209:errorcluster)
        n74 = Bundle By Name(cluster=w211, "Data DVR"=w196, "Sweep Data Cluster"=w204, "Scan names"=w198) -> (w210:T6)
        n75 = call <vilib>:"Add State(s) to Queue__jki_lib_state_machine.vi"("State(s) in (\"\")"=w217) -> ("States Out"=w216:string)  [unwired: 14 in]
      }
      frame "LOAD: empty" {
        # "Your code here.\n(You can make a copy of, or modify, this frame)"
        n76 = call <vilib>:"Add State(s) to Queue__jki_lib_state_machine.vi"("State(s) in (\"\")"=w221) -> ("States Out"=w220:string)  [unwired: 14 in]
      }
      frame "---------- VISUALIZE ----------" {
        # "Template Separator\n(You can make a copy of, or modify, this frame)"
        n77 = call <vilib>:"Add State(s) to Queue__jki_lib_state_machine.vi"("State(s) in (\"\")"=w225) -> ("States Out"=w224:string)  [unwired: 14 in]
      }
      frame "VISUALIZE: Initialize Cursor Graph" {
        # "Template Separator\n(You can make a copy of, or modify, this frame)"
        n78 = Unbundle By Name(w241) -> ("Sweep Data Cluster.Vfast"=w233:dbl[][], "Sweep Data Cluster.Vslow"=w234:dbl[])  [unwired: 1 out]
        n79 = local read "Scan names"() -> (w232:string[])
        n80 = Transpose 2D Array(2D array=w233) -> (transposed array=w240:dbl[][])
        n81 = for {
          tunnel: w240 -> [w249] mode=indexing
          tunnel: [w250] -> _ mode=indexing
          tunnel: w234 -> [w246]
          shift-right: [w247] -> w237
          shift-left: dbl[] [] -> [w248]
          shift-right: [w245] -> w236
          shift-left: dbl[] [] -> [w244]
          n82 = Build Array (concatenate)(w248, w249) -> (w247:dbl[])
          n83 = Build Array (concatenate)(w244, w246) -> (w245:dbl[])
          n84 = Bundle(w249, "Vslow"=w246) -> (w250:cluster{dbl[], "Vslow":dbl[]})  [unwired: 1 in]
        }
        n85 = Index Array(array=w232, index #2=1 ("index")) -> (element #1=w230:string, element #2=w229:string)  [unwired: 1 in]
        n86 = property on="Cursor Graph" class="XYGraph (strict)"(error in=w227, "XScale.NameLbl.Text"=w230) -> (error out=w228:errorcluster)  [unwired: 1 in, 1 out]
        n87 = property on="Cursor Graph" class="XYGraph (strict)"(error in=w228, "YScale.NameLbl.Text"=w229) -> (error out=w226:errorcluster)  [unwired: 1 in, 1 out]
        n88 = Bundle(w237, w236) -> (→"Cursor Graph":cluster{dbl[], dbl[]})  [unwired: 1 in]
        n89 = call <vilib>:"Add State(s) to Queue__jki_lib_state_machine.vi"("State(s) in (\"\")"=w243) -> ("States Out"=w242:string)  [unwired: 14 in]
      }
      frame "VISUALIZE: Initialize Color Tables" {
        # "#TODO:"
        # "Set color tables"
        # "Template Separator\n(You can make a copy of, or modify, this frame)"
        n90 = Reverse 1D Array(array="color scale") -> (reversed array=w253:u32[])
        n91 = call <userlib>:"Make Color Table.vi"("Array"=w253) -> ("Color Tbl"=w251:u32[])  [unwired: 1 in, 3 out]
        n92 = property on="2term Intensity" class="IntGraph (strict)"("Color Table"=w251) -> ()  [unwired: 2 in, 2 out]
        n93 = call <vilib>:"Add State(s) to Queue__jki_lib_state_machine.vi"("State(s) in (\"\")"=w257) -> ("States Out"=w256:string)  [unwired: 14 in]
      }
      frame "VISUALIZE: Apply SG Filter" {
        # "NOT IMPLEMENTED YET\n#TODO: this"
        # "Template Separator\n(You can make a copy of, or modify, this frame)"
        n94 = call <vilib>:"Add State(s) to Queue__jki_lib_state_machine.vi"("State(s) in (\"\")"=w261) -> ("States Out"=w260:string)  [unwired: 14 in]
      }
      frame "VISUALIZE: Cursor Things" {
        # "trash if this all gets put into In-place element structure"
        # "#TODO: work out this state logic, for now just repeat\n'case 3' cursor things and graph something"
        # "Template Separator\n(You can make a copy of, or modify, this frame)"
        n95 = Unbundle By Name(w263) -> ("Sweep Data Cluster.Vfast"=w270:dbl[][], "Sweep Data Cluster.Vslow"=w269:dbl[], "Sweep Data Cluster.Vslowest"=w268:dbl[])
        n96 = disable-structure shown="Enabled" {
          disable-tunnel: w270 -> [w287 _]
          disable-tunnel: w269 -> [w286 _]
          disable-tunnel: w268 -> [w285 _]
          disable-tunnel: [w284 _] -> w267
          disable-tunnel: [w283 _] -> w266
          disable-tunnel: [w282 _] -> w265
          disable-tunnel: [w281 _] -> w264
          frame Disabled {
            n97 = Index Array(array=w285) -> (element=w275:dbl, index=w277:i32)
            n98 = Array Size(array=w285) -> (size(s)=w280:i32)
            n99 = call "DataVIS_Get_Cursor_Indices.vi"("Vslow"=w286, "Vfast"=w287) -> ("Slow Indices"=w282:dbl[], "Slow Index (Cursor Y)"=w283:dbl, "Fast Index (Cursor X) (IDK why it's an array)"=w284:dbl[], "Raw Cursor Position"=w281:T7, "Cursor Graph"=w278:refnum<vi>)  [unwired: 4 in, 1 out]
            n100 = Decrement(x=w280) -> (x-1=w279:i32)
            n101 = Unbundle By Name(w281) -> ("Y"=w274:dbl)  [unwired: 1 out]
            n102 = property on="Property Node" class="Slide (strict)"("Scale.Maximum"=w279) -> (reference=w276:refnum<vi>)  [unwired: 1 in, 2 out]
          }
          frame Enabled {
          }
        }
        n103 = disable-structure shown="Enabled" {
          frame Disabled {
            n104 = local read "side points 4Ttemp"() -> (w297:i32)
            n105 = local read "side points 2Ttemp"() -> (w298:i32)
            n106 = local read "side points 2T 2"() -> (w299:i32)
            n107 = local read "side points 4T 2"() -> (w296:i32)
            n108 = Not Equal?(x=w297, y=w296) -> (x != y?=w295:bool)
            n109 = Not Equal?(x=w299, y=w298) -> (x != y?=w294:bool)
            n110 = Or(x=w295, y=w294) -> (x .or. y?=w293:bool)
            n111 = Select(t=2, s=w293, f=3) -> (s? t:f=w288:i32)
            n112 = Select(t=4, f=w288) -> (s=w291:bool)  [unwired: 1 out]
          }
          frame Enabled {
          }
        }
        n113 = Bundle By Name(cluster=w263, "Cursor Info.Fast Index"=w267, "Cursor Info.Slow Index"=w266, "Cursor Info.Slow Indices"=w265, "Cursor Info.Raw Cursor Position"=w264) -> (w262:T6)
        n114 = call <vilib>:"Add State(s) to Queue__jki_lib_state_machine.vi"("State(s) in (\"\")"=w273) -> ("States Out"=w272:string)  [unwired: 14 in]
      }
      frame "VISUALIZE: Graph Something" {
        # "#TODO: if it's slow, keep the main looping INSIDE this"
        n115 = Unbundle By Name(w306) -> ("Data DVR"=w303:refnum<data-value>, "Scan names"=w309:string[], "Cursor Info.Slow Index"=w302:dbl, "Sweep Data Cluster.Comments"=→"Comments":string)
        n116 = in-place {
          in-place-border: w302 -> [w344]
          in-place-border: w309 -> [w343]
          in-place-border: w306 -> [w311]
          in-place-border: [w342] -> w307
          in-place-border: w308 -> [w313]
          in-place-border: [w310] -> w301
          # "Line Cuts"
          # "update cursor"
          # "Offset and step of fast vals"
          # "Decimate it"
          # "Select an AvsB curve"
          n117 = in-place-dvr #1(w303) -> (w331:T4)  [unwired: 1 out]
          n118 = call "ZDataVIS_Select_Intensity.vi"("B"="Z Axis", "A"="X Axis", "error in (no error)"=w313, "Slow Index (Row)"=w344, "Slowest Index (Page)"="Field/Temperature", "Big Ol Array IN"=w331) -> ("error out"=w335:errorcluster, "Intensity Info OUT"=w330:cluster{dbl[], dbl[]}[])  [unwired: 4 in]
          n119 = Index Array(array=w343, index="Z Axis") -> (element=w338:string)
          n120 = call "ZDataVIS_ScaleSelect.vi"("Manual CTLs"="Manual CTLs", "Auto CTLs"="Auto CTLs", "error in (no error)"=w335, "X Scale Selection 2"="X Scale Selection", "Intensity Info IN"=w330) -> ("error out"=w334:errorcluster, "X Step Info"=w327:cluster{"X Low":dbl, "X High":dbl, "X Step":dbl}, "Intensity InfoOUT"=w326:cluster{dbl[], dbl[]}[])  [unwired: 4 in]
          n121 = Index Array(array=w326) -> (element=→"XY Graph":cluster{dbl[], dbl[]})  [unwired: 1 in]
          n122 = call "ZDataVIS_Decimate+Fill_Intensity_Plot.vi"("Voffset -2T"="Voffset -2T", "error in (no error)"=w334, "fake point value"="Fake Point Value", "Step Info"=w327, "X and Y Arrays to decimate"=w326) -> ("error out"=w328:errorcluster, "Decimated X values"=w318:dbl[], "Arr of Y arrays (intensity info)"=w337:dbl[][])  [unwired: 4 in]
          n123 = control-ref of="2term Intensity"() -> (w315:refnum<vi>)
          n124 = call "ZDataVIS_XY_Offset+Mult.vi"("Voffset -2T"="Voffset -2T", "error in (no error)"=w328, "X Step Info"=w327, "State Wire IN"=w311) -> ("error out"=w324:errorcluster, "Y Offset+Mult"=w320:cluster{"Offset X Low":dbl, "X Step":dbl}, "X Offset+Mult"=w321:cluster{"Offset X Low":dbl, "X Step":dbl}, "State Wire OUT"=w322:T6)  [unwired: 4 in]
          n125 = Transpose 2D Array(2D array=w337) -> (transposed array=w319:dbl[][])
          "2term Intensity" <- w319
          n126 = call "ZDataVIS_LineCuts.vi"("Intensity Plot"=w315, "e^2/h?"="e^2/h?", "error in (no error)"=w324, "Decimated X values"=w318, "Arr of Y arrays (intensity info)"=w319, "State Wire IN"=w322) -> ("error out"=w323:errorcluster, "X line cut"=→"X line cut":cluster{dbl[], dbl[]}, "Y line cut"=→"Y line cut":cluster{"Vfast":dbl[], dbl[]}, "State Wire OUT"=w310:T6)  [unwired: 2 in]
          n127 = call "ZDataVIS_Configure_Intensity_Plot.vi"("Scan Name"=w338, "error in (no error)"=w323, "Y Offset and Multiplier"=w320, "X Offset and Multiplier"=w321, "IntensityGraph in"=w315) -> ("error out"=w342:errorcluster)  [unwired: 6 in]
          n128 = in-place-dvr #1(w331) -> ()  [unwired: 2 out]
        }
        n129 = call <vilib>:"Add State(s) to Queue__jki_lib_state_machine.vi"("State(s) in (\"\")"=w305) -> ("States Out"=w304:string)  [unwired: 14 in]
      }
    }
  }
